vi "JointImage.vi"(0 "文件根路径":path=path "D:/做的项目/航天测量/拼接", 1 "Y方向图像个数":i32=6, 2 "降采样倍数":i32=4, 3 "X方向图像个数":i32=6, 4 "单张图片大小":i32=4096) -> (5 "JointImage Out":T1)   [LabVIEW 2018]
uses:
  <vilib>/vision/Image Controls.llb/IMAQ Image.ctl
  <vilib>/vision/NI_Vision_Development_Module.lvlib
panel:
  out "进度":dbl(slide) scale=0.0..1.0
  out "子图像":T1(plugin-control)
  out "拼接图":T1(plugin-control)
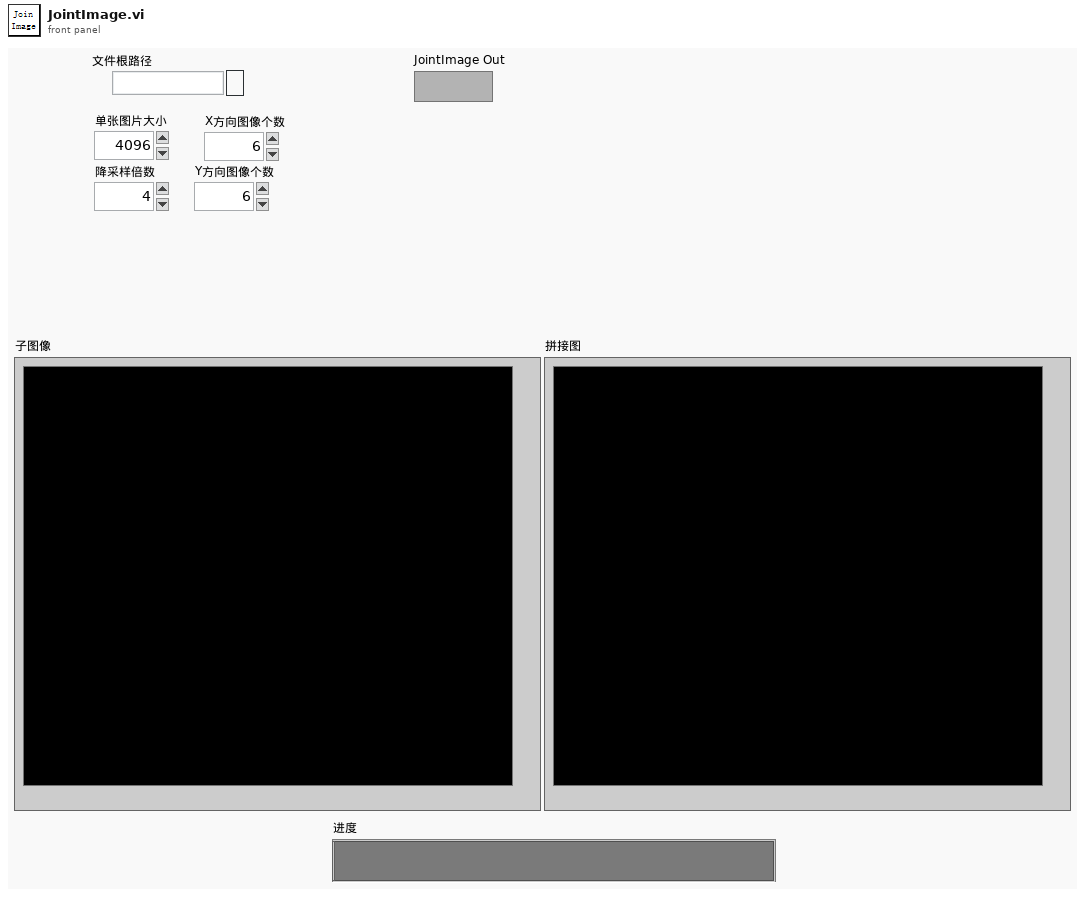
[diagram p1: front panel]
types:
  T1 = typedef "IMAQ Image.ctl" = refnum<image>
  T2 = typedef "Image Type" = u32
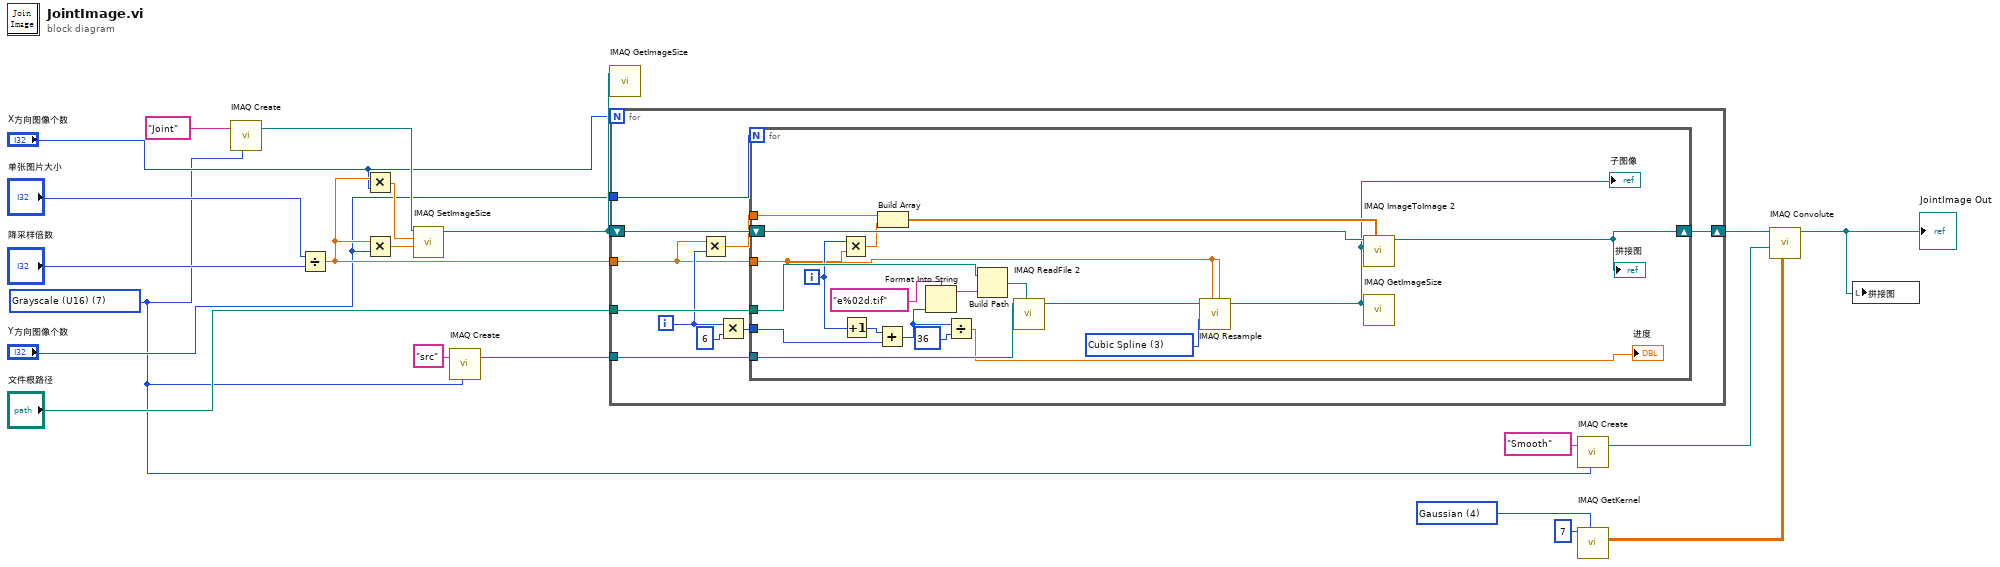
[diagram p0: block diagram]
diagram:
  w6 = u16 4 items=["Gradient"=1, "Laplacian"=2, "Smoothing"=3, "Gaussian"=4] ("Kernel Family")
  w3 = T2 7 items=["Grayscale (U8)", "Grayscale (I16)", "Grayscale (SGL)", "Complex (CSG)", "RGB (U32)", "HSL (U32)", "RGB (U64)", "Grayscale (U16)"] ("Image Type")
  n1 = call "IMAQ Create"("Image Name"="Joint", "Image Type"=w3) -> ("New Image"=w20:T1)  [unwired: 3 in, 1 out]
  n2 = Divide(x="单张图片大小", y="降采样倍数") -> (x/y=w12:dbl)
  n3 = Multiply(x=w12, y="X方向图像个数") -> (x*y=w13:dbl)
  n4 = Multiply(x=w12, y="Y方向图像个数") -> (x*y=w11:dbl)
  n5 = call "IMAQ SetImageSize"("Y Resolution"=w11, "X Resolution"=w13, "Image"=w20) -> ("Image Out"=w14:T1)  [unwired: 2 in, 1 out]
  n6 = call "IMAQ Create"("Image Name"="src", "Image Type"=w3) -> ("New Image"=w16:T1)  [unwired: 3 in, 1 out]
  n7 = call "IMAQ GetImageSize"("Image"=w14) -> ()  [unwired: 3 in, 3 out]
  n8 = for {
    N: "X方向图像个数" -> [_]
    tunnel: w16 -> [w31]
    tunnel: "文件根路径" -> [w30]
    shift-right: [w29] -> w8
    shift-left: w14 -> [w28]
    tunnel: w12 -> [w24]
    tunnel: "Y方向图像个数" -> [w22]
    i -> [w25]
    n9 = Multiply(x=w24, y=w25) -> (x*y=w23:dbl)
    n10 = Multiply(x=w25, y=6) -> (x*y=w26:i32)
    n11 = for {
      N: w22 -> [_]
      tunnel: w31 -> [w51]
      tunnel: w30 -> [w50]
      shift-right: [w32] -> w29
      shift-left: w28 -> [w46]
      tunnel: w26 -> [w45]
      tunnel: w23 -> [w33]
      tunnel: w24 -> [w36]
      i -> [w44]
      w37 = u32 3 items=["Zero Order", "Bi-Linear", "Quadratic", "Cubic Spline"] ("Interpolation Type")
      n12 = Multiply(x=w44, y=w36) -> (x*y=w34:dbl)
      n13 = Increment(x=w44) -> (x+1=w42:i32)
      n14 = Add(x=w42, y=w45) -> (x+y=w41:i32)
      n15 = Build Array(w33, w34) -> (w43:dbl[])
      n16 = Format Into String(format string="e%02d.tif" ("格式字符串"), w41) -> (resulting string=w49:string)  [unwired: 2 in, 1 out]
      n17 = Divide(x=w41, y=36) -> (x/y=→"进度":dbl)
      n18 = Build Path(base path=w50, name or relative path=w49) -> (appended path=w47:path)
      n19 = call "IMAQ ReadFile 2"("File Path"=w47, "Image"=w51) -> ("Image Out"=w38:T1)  [unwired: 5 in, 4 out]
      n20 = call "IMAQ Resample"("X Resolution"=w36, "Y Resolution"=w36, "Interpolation Type"=w37, "Image Src"=w38) -> ("Image Dst Out"=w35:T1)  [unwired: 6 in, 1 out]
      "子图像" <- w35
      n21 = call "IMAQ ImageToImage 2"("Offset Left/Top"=w43, "Image Src (Small)"=w35, "Image Src (Large)"=w46) -> ("Image Dst Out"=w32:T1)  [unwired: 7 in, 1 out]
      "拼接图" <- w32
      n22 = call "IMAQ GetImageSize"("Image"=w35) -> ()  [unwired: 3 in, 3 out]
    }
  }
  n23 = call "IMAQ Create"("Image Name"="Smooth", "Image Type"=w3) -> ("New Image"=w2:T1)  [unwired: 3 in, 1 out]
  n24 = call "IMAQ GetKernel"("Kernel Family"=w6, "Kernel Size (3,5,...)"=7) -> ("Kernel"=w7:sgl[][])  [unwired: 6 in, 3 out]
  n25 = call "IMAQ Convolute"("Kernel"=w7, "Image Dst"=w2, "Image Src"=w8) -> ("Image Dst Out"=w1:T1)  [unwired: 7 in, 1 out]
  "JointImage Out" <- w1
  n26 = local write "拼接图"(w1) -> ()
